vi "LinkDeviceReadWrite.vi"() -> (2 "Table Control":string[][](table))   [LabVIEW 2019]
uses:
  C:/Users/chrismadlax/Desktop/LabVIEW-BLE-Driver/BLELib.dll
  BLELib.dll
panel:
  in  "LinkDevice":bool
  out "INIT":bool
  in  "RAWAddress":u64=69987970987151
  in  "CharacteristicUUID":string="19b10001-e8f2-537e-4f6c-d104768a1214"
  out "Numeric":i32
  out "Result":string
  in  "Boolean":bool
  out "ServicesUUIDs Value":string
  out "Pair Result":string
  # "Arduino BLE 33 board RAWaddress"
  # "A4:DA:32:0D:F5:E2"
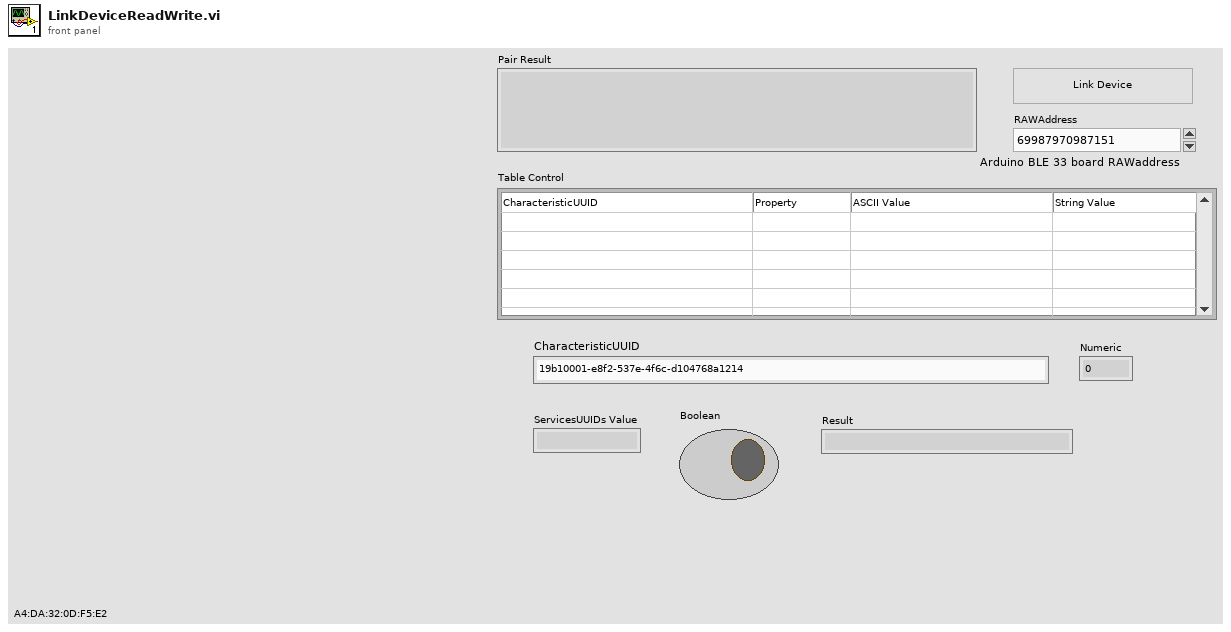
[diagram p1: front panel]
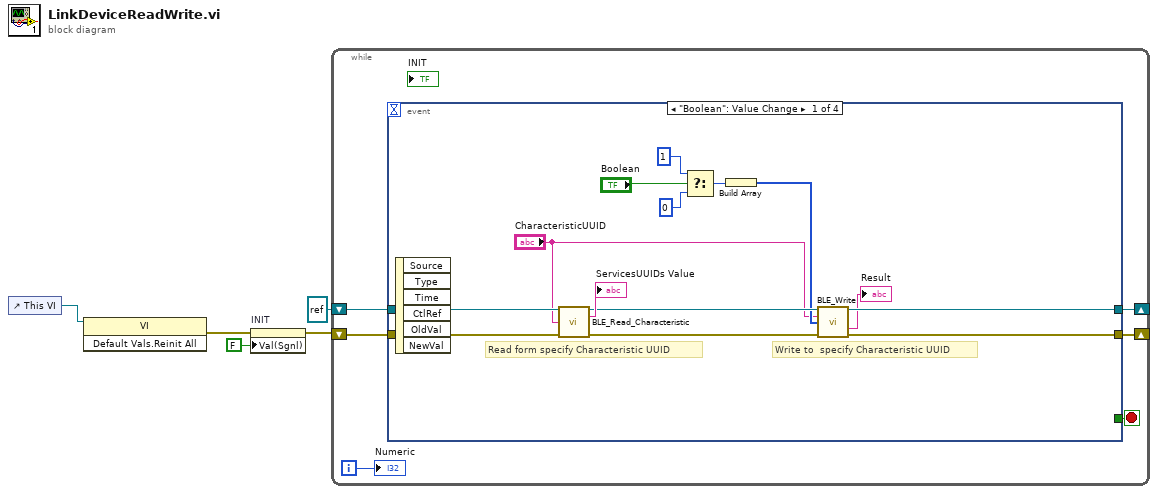
[diagram p0: block diagram]
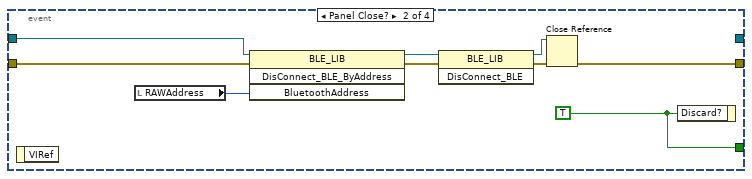
[diagram p2: hidden frame]
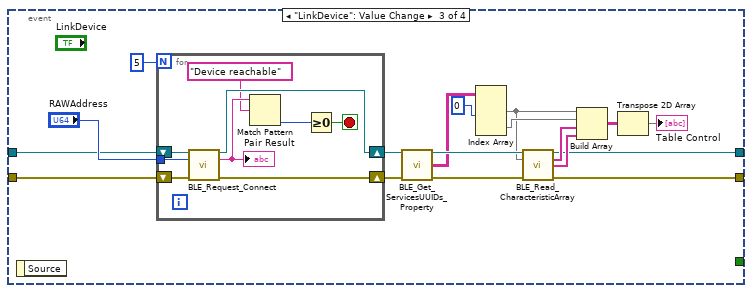
[diagram p3: hidden frame]
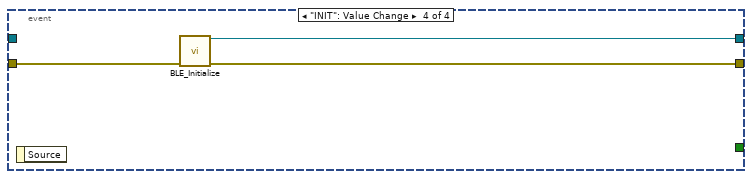
[diagram p4: hidden frame]
diagram:
  n1 = control-ref of="This VI"() -> (w1:refnum<vi>)
  n2 = invoke class="VI" method="Default Vals.Reinit All"(reference=w1) -> (error out=w2:errorcluster)  [unwired: 2 in, 2 out]
  n3 = property on="INIT" class="Bool (strict)"(error in=w2, "Val(Sgnl)"=FALSE ("Value (Signaling)")) -> (error out=w5:errorcluster)  [unwired: 1 in, 1 out]
  n4 = while {
    shift-right: [w8] -> _
    shift-left: refnum<k24> refnum (".NET Refnum out") -> [w11]
    shift-right: [w9] -> _
    shift-left: w5 -> [w10]
    i -> [w7]
    stop <- w6 stop-if-true
    n5 = event shown="[0] \"Boolean\": Value Change" {
      selector: _ -> [_ _ _ _]
      dyn-events: _ -> [_ _ _ _]
      timeout: _ -> [_ _ _ _]
      tunnel: w11 -> [w25 w27 w38 _]
      tunnel: w10 -> [w24 w29 w37 w64]
      tunnel: [w21 w28 w36 w63] -> w9
      tunnel: [w19 _ w35 w62] -> w8
      tunnel: [_ w34 _ _] -> w6
      event "Boolean": Value Change {
        # "Write to  specify Characteristic UUID"
        # "Read form specify Characteristic UUID"
        n6 = event-data() -> ()  [unwired: 1 in, 6 out]
        n7 = call "BLE_Read_Characteristic.vi"(".NET Refnum in"=w25, "CharacteristicUUID"="CharacteristicUUID", "error in (no error)"=w24) -> (".NET Refnum out"=w20:refnum<k24>, "ServicesUUIDs Value"=→"ServicesUUIDs Value":string, "error out"=w23:errorcluster)  [unwired: 8 in, 2 out]
        n8 = Select(t=u8 1, s="Boolean", f=u8 0) -> (s? t:f=w16:u8)
        n9 = Build Array(w16) -> (w13:u8[])
        n10 = call "BLE_Write.vi"(".NET Refnum in"=w20, "UUID"="CharacteristicUUID", "WriteByteArray"=w13, "error in (no error)"=w23) -> (".NET Refnum out"=w19:refnum<k24>, "Result"=→"Result":string, "error out"=w21:errorcluster)  [unwired: 9 in]
      }
      event Panel Close? {
        w34 = TRUE ("Discard?")
        n11 = event-data() -> ()  [unwired: 1 in, 1 out]
        n12 = local read "RAWAddress"() -> (w26:u64)
        n13 = invoke class="BLE_LIB" method="DisConnect_BLE_ByAddress"(reference=w27, error in=w29, "BluetoothAddress"=w26) -> (reference out=w33:refnum<k24>, error out=w31:errorcluster)  [unwired: 1 in, 2 out]
        n14 = invoke class="BLE_LIB" method="DisConnect_BLE"(reference=w33, error in=w31) -> (reference out=w32:refnum<k24>, error out=w30:errorcluster)  [unwired: 1 in, 1 out]
        n15 = Close Reference(reference=w32, error in (no error)=w30) -> (error out=w28:errorcluster)
        n16 = event-data("Discard?"=w34) -> ()  [unwired: 1 in, 1 out]
      }
      event "LinkDevice": Value Change {
        n17 = event-data() -> ()  [unwired: 1 in, 1 out]
        n18 = for {
          N: 5 -> [_]
          tunnel: "RAWAddress" -> [w59]
          shift-right: [w57] -> w42
          shift-left: w37 -> [w61]
          shift-right: [w58] -> w41
          shift-left: w38 -> [w60]
          stop <- w53 stop-if-true
          n19 = call "BLE_Request_Connect.vi"(".NET Refnum in"=w60, "BluetoothAddress"=w59, "error in (no error)"=w61) -> (".NET Refnum out"=w58:refnum<k24>, "ConnectBLE"=w56:string, "error out"=w57:errorcluster)  [unwired: 10 in]
          "Pair Result" <- w56
          n20 = Match Pattern(string=w56, regular expression="Device reachable") -> (offset past match=w54:i32)  [unwired: 1 in, 3 out]
          n21 = Greater Or Equal To 0?(x=w54) -> (x >= 0?=w53:bool)
        }
        n22 = call "BLE_Get_ServicesUUIDs_Property.vi"(".NET Refnum in"=w41, "error in (no error)"=w42) -> (".NET Refnum out"=w51:refnum<k24>, "Char Val-Property"=w49:string[][], "error out"=w50:errorcluster)  [unwired: 11 in]
        n23 = Index Array(array=w49, index (col) #1=0 ("disabled index (col)")) -> (element #1=w46:string[], element #2=w47:string[])  [unwired: 3 in]
        n24 = call "BLE_Read_CharacteristicArray.vi"(".NET Refnum in"=w51, "ServicesUUIDs Extract Value"=w46, "error in (no error)"=w50) -> (".NET Refnum out"=w35:refnum<k24>, "ServicesUUIDs ASCII Value"=w43:string[], "ServicesUUIDs Value"=w44:string[], "error out"=w36:errorcluster)  [unwired: 9 in]
        n25 = Build Array(w46, w47, w43, w44) -> (w45:string[][])
        n26 = Transpose 2D Array(2D array=w45) -> (transposed array=→"Table Control":string[][])
      }
      event "INIT": Value Change {
        n27 = event-data() -> ()  [unwired: 1 in, 1 out]
        n28 = call "BLE_Initialize.vi"("error in (no error)"=w64) -> (".NET Refnum out"=w62:refnum<k24>, "error out"=w63:errorcluster)  [unwired: 13 in]
      }
    }
    "Numeric" <- w7
  }
